vi "Get State.vi"(8 "error in":errorcluster, 11 "Instrument in":refnum<class "Instrument.lvclass">) -> (0 "error out":errorcluster, 2 "default state":T1, 3 "Instrument out":refnum<class "Instrument.lvclass">)   [LabVIEW 2017, in "Instrument.lvclass"]
doc: "Retrieves the current state from the state queue. If the queue is empty, then the state will default to the that specified by the user."
uses:
  Instrument.lvclass
  state.ctl
  Instrument.lvclass/Instrument.ctl
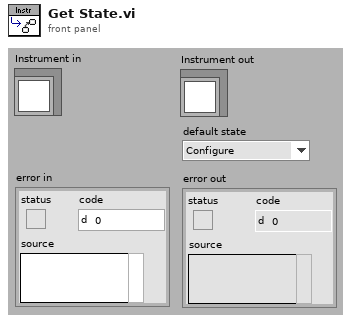
[diagram p1: front panel]
types:
  T1 = typedef "Instrument.lvclass/state.ctl" = enum8{"Configure", "Acquire", "Wait", "Quit", "Handle Error", "NOOP"}
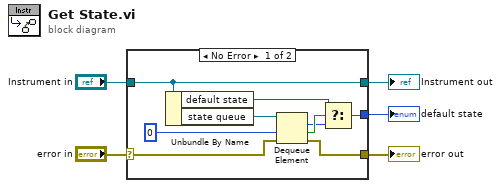
[diagram p0: block diagram]
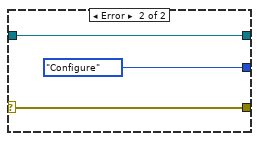
[diagram p2: hidden frame]
diagram:
  n1 = case shown="No Error" "error in" {
    selector: "error in" -> [w7 w17]
    tunnel: [w6 w17] -> w4
    tunnel: [w14 w16] -> w2
    tunnel: "Instrument in" -> [w14 w16]
    tunnel: [w11 state."Configure" ("instr state")] -> w1
    frame No Error {
      n2 = Unbundle By Name(w14) -> ("default state"=w10:T1, "state queue"=w13:refnum<queue>)
      n3 = Dequeue Element(queue=w13, timeout in ms (-1)=0, error in (no error)=w7) -> (element=w8:T1, timed out?=w9:bool, error out=w6:errorcluster)  [unwired: 1 out]
      n4 = Select(t=w10, s=w9, f=w8) -> (s? t:f=w11:T1)
    }
    frame Error {
    }
  }
  "error out" <- w4
  "Instrument out" <- w2
  "default state" <- w1
